vi "pci-6713-6025E-6733(set all analog).vi"(4 "6221 Control":dbl[](array[numeric])=[6.5, 7.0], 5 "Change 6221?":bool, 6 "6733 Control":sgl[](array[numeric])=[8.0, 3.0, 4.0, 0.0, 0.0, 6.46, 6.98, 0.0] format="%.3f", 7 "Change 6733":bool, 8 "6713 Control":sgl[](array[numeric])=[4.6, 0.5, 0.035, 7.35, 10.0, 4.0, 4.0, 2.703] format="%.3f", 9 "Change 6713?":bool=TRUE) -> (0 "Voltage limit (+-10V)":string[](array[string])=["OK ", "OK ", "OK ", "OK ", "OK ", "OK ", "OK ", "OK "], 1 "6733 Status":string="PCI-6733 OK", 2 "Voltage limit (+-10V)":string[](array[string])=["OK ", "OK ", "OK ", "OK ", "OK ", "OK ", "OK ", "OK "], 3 "6713 Status":string="PCI-6713 OK")   [LabVIEW 2013]
uses:
  AO Update Channel (scaled value).vi
  Instance           4 43Saved   pci-6713-6025E-6733(set all analog) .vi
  Instance           5 43Saved   pci-6713-6025E-6733(set all analog) .vi
  <vilib>/DAQmx/write.llb/DAQmx Write (Analog DBL 1Chan 1Samp).vi
panel:
  in  "Case Constant\n(See Context Help) 4":bool
  in  "Case Constant\n(See Context Help) 3":bool
  in  "Case Constant\n(See Context Help) 2":bool
  in  "Change 6025?":bool
  in  "Case Constant\n(See Context Help)":bool
  out "6733 Status 2":string="PCI-6733 OK"
  in  "6733 Control 2":sgl[](array[numeric])=[8.0, 3.0, 4.0, 0.0, 0.0, 6.46, 6.98, 0.0] format="%.3f"
  out "Voltage limit (+-10V) 2":string[](array[string])=["OK ", "OK ", "OK ", "OK ", "OK ", "OK ", "OK ", "OK "]
  out "Array 3":sgl[](array[numeric])=[8.0, 3.0, 4.0, 0.0, 0.0, 6.46, 6.98, 0.0]
  out "error out":errorcluster
  in  "Change 87Sr 6733":bool
  in  "87Sr 6733 Control":sgl[](array[numeric])=[8.0, 3.0, 4.0, 0.0, 0.0, 6.46, 6.98, 0.0] format="%.3f"
  out "87Sr Voltage limit (+-10V)":string[](array[string])=["OK ", "OK ", "OK ", "OK ", "OK ", "OK ", "OK ", "OK "]
  out "Array 2":sgl[](array[numeric])=[8.0, 3.0, 4.0, 0.0, 0.0, 6.46, 6.98, 0.0]
  out "Array":sgl[](array[numeric])=[8.0, 3.0, 4.0, 0.0, 0.0, 6.46, 6.98, 0.0]
  out "Voltage Limit (":string[](array[string])=["OK ", "OK "]
  in  "6025 Control":sgl[](array[numeric])=[-0.15, 0.1] format="%.3f"
  out "6025 Status":string="PCI-6025E OK"
  # "0..satabs offset for imaging"
  # "1... MOT power"
  # "2....MOT Jump Power"
  # "3....GENERAL PARAMETER: PAS AOM"
  # "4... GenPAram: offset lock"
  # "5....Vset for Lambda (0 to 10V)(pos for FET lock)"
  # "The DC supply\nvoltage for the\nZOS was 14.1 V"
  # "6....satabs offset for MOT"
  # "7.... satabs offset for cooling"
  # "0.....422 image AOM"
  # "PCI-6025E is NOT functional for Neutral Atoms.\nIt has been disabled in the block diagram, so\nchanging any of these values will not affect \nanything."
  # "1.....openr"
  # "Right now, put in units of \nvolts.  Freq to voltage \nconversion later."
  # "0.....100MHz Red MOT AOM (ZOS100) MHZ"
  # "1..... Power Control on  Red MOT AOM 5V full"
  # "dimage1 6.46V = 51.81MHz"
  # "dmot 6.980V = 35.50MHz"
  # "0.. Image AOM VCO (5V=41.5)"
  # "0..MOT AOM VCO (5V=41.5)"
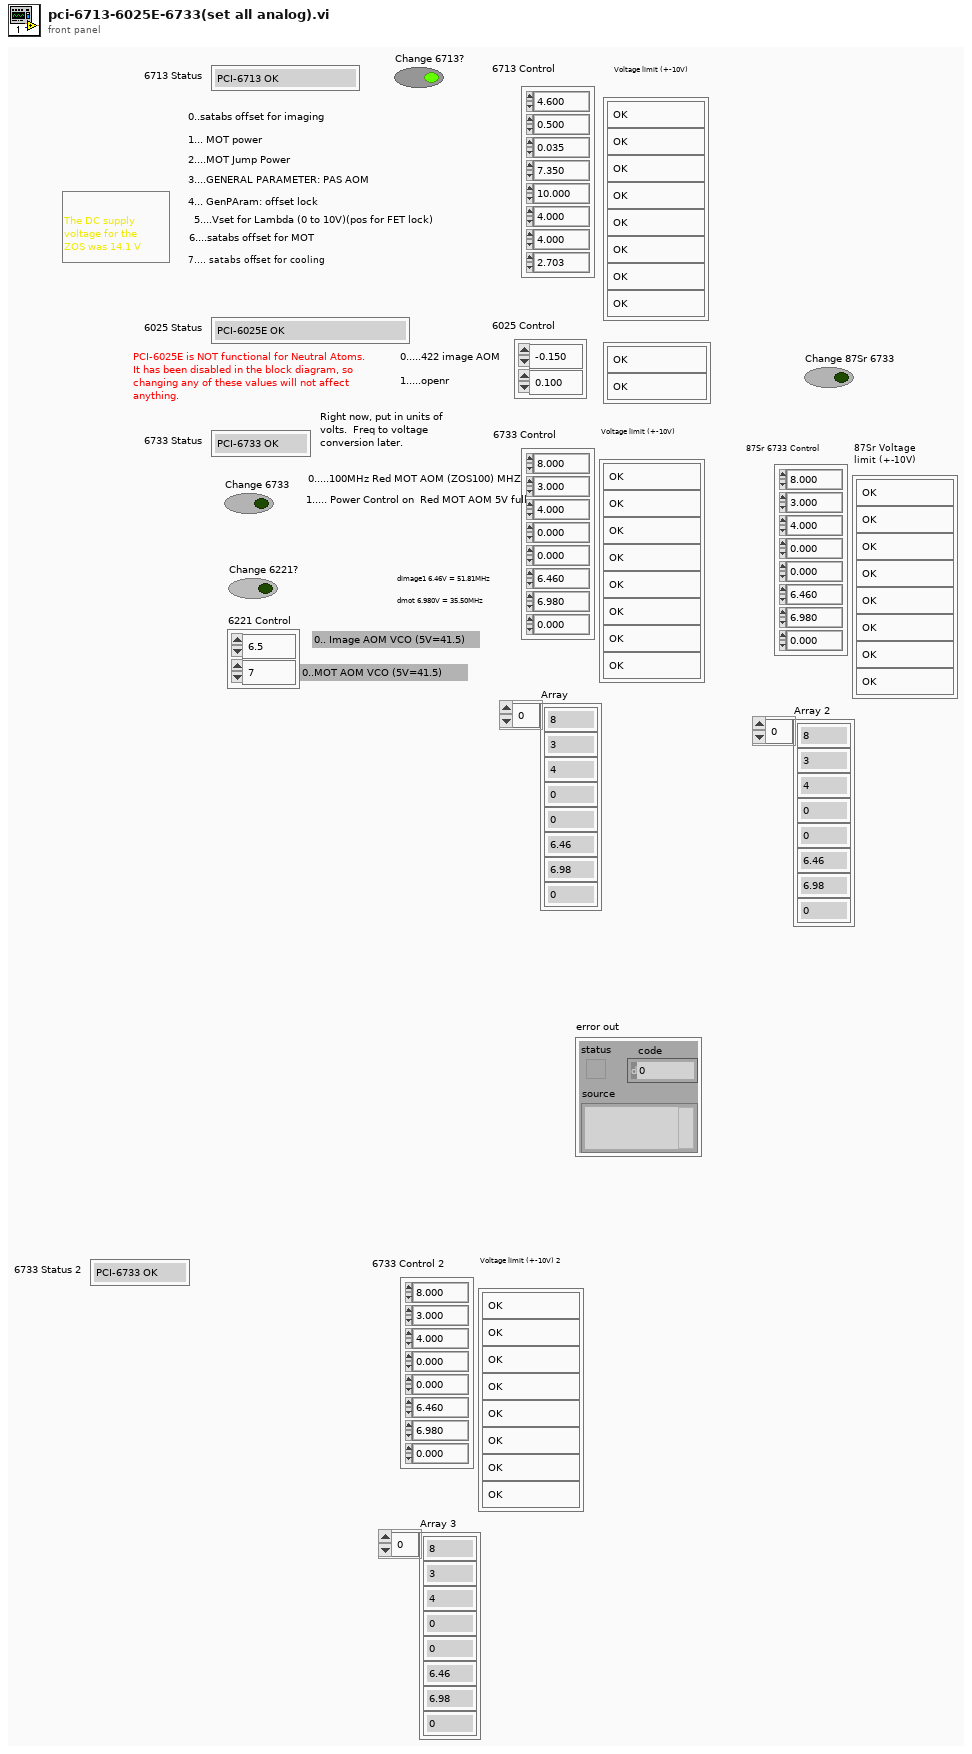
[diagram p1: front panel]
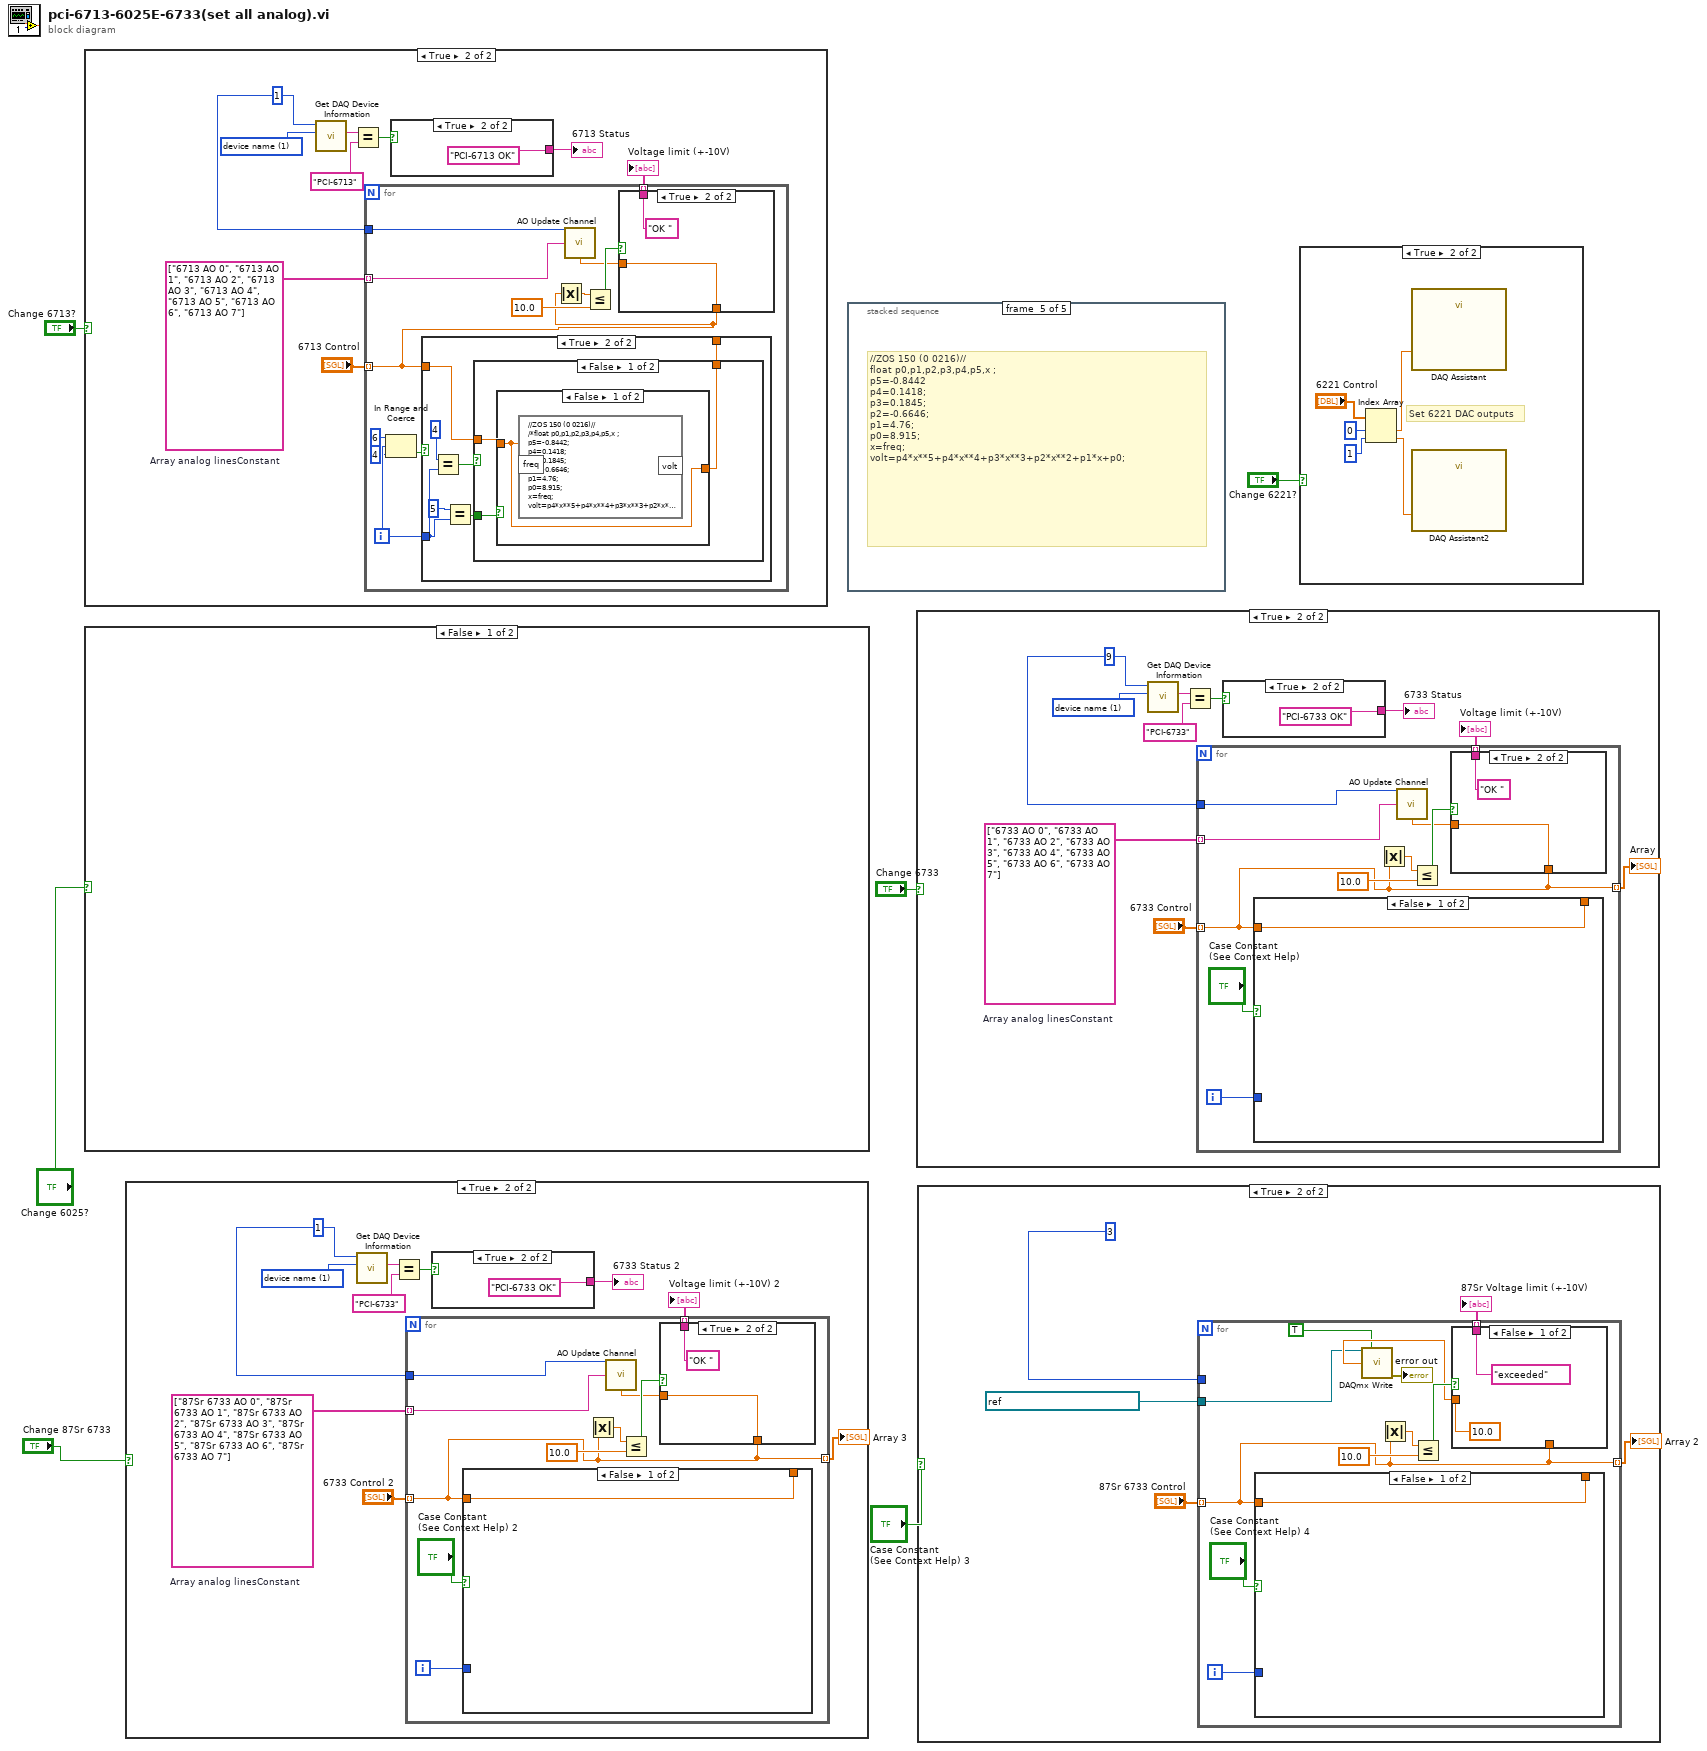
[diagram p0: block diagram]
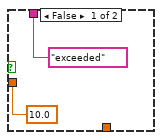
[diagram p3: hidden frame]
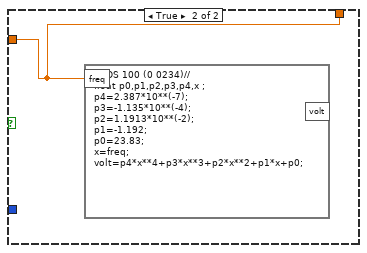
[diagram p4: hidden frame]
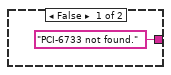
[diagram p5: hidden frame]
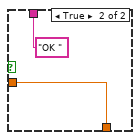
[diagram p7: hidden frame]
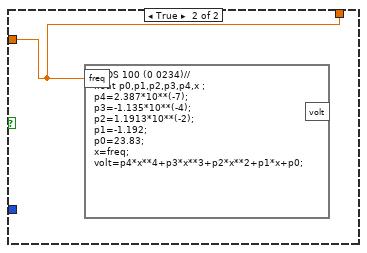
[diagram p8: hidden frame]
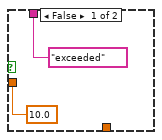
[diagram p11: hidden frame]
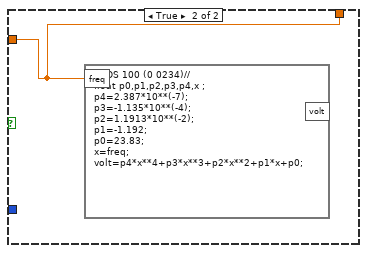
[diagram p12: hidden frame]
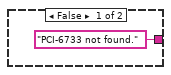
[diagram p13: hidden frame]
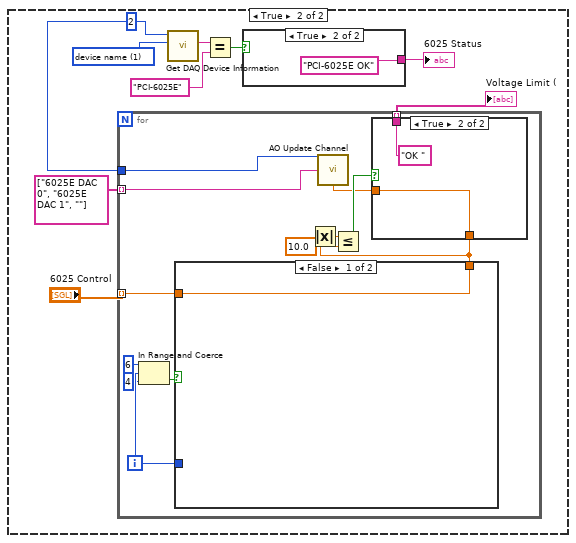
[diagram p14: hidden frame]
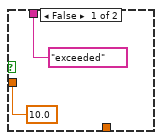
[diagram p15: hidden frame]
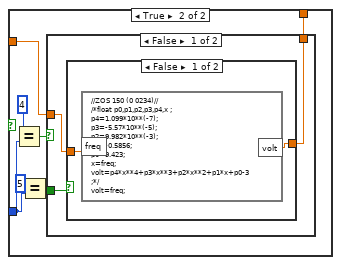
[diagram p16: hidden frame]
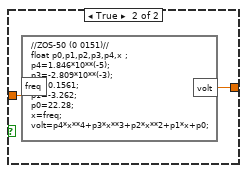
[diagram p17: hidden frame]
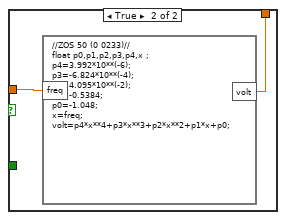
[diagram p18: hidden frame]
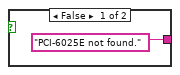
[diagram p19: hidden frame]
diagram:
  n1 = case shown="True" "Change 6713?" {
    frame False {
    }
    frame True {
      w7 = tag[] ["6713 AO 0", "6713 AO 1", "6713 AO 2", "6713 AO 3", "6713 AO 4", "6713 AO 5", "6713 AO 6", "6713 AO 7"]  # Array analog linesConstant
      w15 = u32 1 items=["NI-DAQ version", "device name", "base address", "data transfer mode for analog input", "data transfer mode for analog output group 1", "data transfer mode for analog output group 2", "data transfer mode for GPCTR 0", "data transfer mode for GPCTR 1", "data transfer mode for digital I/O group 1", "data transfer mode for digital I/O group 2", "device type code", "DMA A level", "DMA B level", "DMA C level", "interrupt A level", "interrupt B level", "reserved", "lpt device mode", "DAQCard-700 counter 1 source", "interrupt generation mode", "device state during suspend mode", "computer name", "serial number", "counter type"] ("information type")
      w10 = u32 1 ("task ID or device")
      n2 = call "Get DAQ Device Information.vi"("information type"=w15, "task ID or device"=w10) -> ("information string"=w14:string)  [unwired: 7 in, 2 out]
      n3 = Equal?(x=w14, y="PCI-6713") -> (x = y?=w12:bool)
      n4 = for {
        tunnel: w10 -> [w27]
        tunnel: "6713 Control" -> [w16] mode=indexing
        tunnel: w7 -> [w26] mode=indexing
        tunnel: [w17] -> w8 mode=indexing
        i -> [w25]
        n5 = In Range and Coerce(upper limit=6, x=w25, lower limit=4) -> (In Range?=w22:bool)  [unwired: 1 out]
        n6 = case shown="True" w22 {
          tunnel: w16 -> [w32 w34]
          tunnel: [w32 w33] -> _
          tunnel: w25 -> [_ w37]
          frame False {
          }
          frame True {
            n7 = Equal?(x=4, y=w37) -> (x = y?=w38:bool)
            n8 = Equal?(x=5, y=w37) -> (x = y?=w35:bool)
            n9 = case shown="False" w38 {
              tunnel: w35 -> [w42 _]
              tunnel: w34 -> [w41 w46]
              tunnel: [w40 w46] -> w33
              frame False {
                n10 = case shown="False" w42 {
                  tunnel: w41 -> [w43 w45]
                  tunnel: [w43 w44] -> w40
                  frame False {
                    n11 = formula code="//ZOS 150 (0 0216)//\n/*float p0,p1,p2,p3,p4,p5,x ;\np5=-0.8442;\np4=0.1418;\np3=0.1845;\np2=-0.6646;\np1=4.76;\np0=8.915;\nx=freq;\nvolt=p4*x**5+p4*x**4+p3*x**3+p2*x**2+p1*x+p0;\n*/\nvolt=freq;"("freq"=w43) -> ()  [unwired: 1 out]
                  }
                  frame True {
                    n12 = formula code="//ZOS 100 (0 0214)//\nfloat p0,p1,p2,p3,p4,x ;\np4=6.457*10**(-7);\np3=-2.117*10**(-4);\np2=2.473*10**(-2);\np1=-0.9844;\np0=11.55;\nx=freq;\nvolt=p4*x**4+p3*x**3+p2*x**2+p1*x+p0;"("freq"=w45) -> ("volt"=w44:dbl)
                  }
                }
              }
              frame True {
                n13 = formula code="//ZOS 150 (0 0234)//\nfloat p0,p1,p2,p3,p4,x ;\np4=1.099*10**(-7);\np3=-5.57*10**(-5);\np2=9.982*10**(-3);\np1=-0.5866;\np0=9.423;\nx=freq;\nvolt=p4*x**4+p3*x**3+p2*x**2+p1*x+p0;"("freq"=w46) -> ()  [unwired: 1 out]
              }
            }
          }
        }
        n14 = Absolute Value(x=w16) -> (abs(x)=w21:sgl)
        n15 = Less Or Equal?(x=w21, y=10.0) -> (x <= y?=w19:bool)
        n16 = case shown="True" w19 {
          tunnel: w16 -> [_ w31]
          tunnel: [10.0 w31] -> w18
          tunnel: ["exceeded" ("String") "OK " ("String")] -> w17
          frame False {
          }
          frame True {
          }
        }
        n17 = call-poly "AO Update Channel.vi"("value"=w18, "channel (0)"=w26, "device"=w27) -> ()
      }
      "Voltage limit (+-10V)" <- w8
      n18 = case shown="True" w12 {
        tunnel: ["PCI-6713 not found." "PCI-6713 OK"] -> w11
        frame False {
        }
        frame True {
        }
      }
      "6713 Status" <- w11
    }
  }
  n19 = case shown="False" "Change 6025?" {
    frame False {
    }
    frame True {
      w57 = u32 1 items=["NI-DAQ version", "device name", "base address", "data transfer mode for analog input", "data transfer mode for analog output group 1", "data transfer mode for analog output group 2", "data transfer mode for GPCTR 0", "data transfer mode for GPCTR 1", "data transfer mode for digital I/O group 1", "data transfer mode for digital I/O group 2", "device type code", "DMA A level", "DMA B level", "DMA C level", "interrupt A level", "interrupt B level", "reserved", "lpt device mode", "DAQCard-700 counter 1 source", "interrupt generation mode", "device state during suspend mode", "computer name", "serial number", "counter type"] ("information type")
      w52 = u32 2 ("task ID or device")
      n20 = for {
        tunnel: w52 -> [w70]
        tunnel: "6025 Control" -> [w64] mode=indexing
        tunnel: tag[] ["6025E DAC 0", "6025E DAC 1", ""] ("Array analog linesConstant") -> [w69] mode=indexing
        tunnel: [w58] -> w50 mode=indexing
        i -> [w68]
        n21 = In Range and Coerce(upper limit=6, x=w68, lower limit=4) -> (In Range?=w65:bool)  [unwired: 1 out]
        n22 = case shown="False" w65 {
          tunnel: w64 -> [w75 w77]
          tunnel: [w75 w76] -> w63
          tunnel: w68 -> [_ w80]
          frame False {
          }
          frame True {
            n23 = Equal?(x=4, y=w80) -> (x = y?=w81:bool)
            n24 = Equal?(x=5, y=w80) -> (x = y?=w78:bool)
            n25 = case shown="False" w81 {
              tunnel: w78 -> [w85 _]
              tunnel: w77 -> [w84 w91]
              tunnel: [w83 w90] -> w76
              frame False {
                n26 = case shown="False" w85 {
                  tunnel: w84 -> [w87 w89]
                  tunnel: [w86 w88] -> w83
                  frame False {
                    n27 = formula code="//ZOS 150 (0 0234)//\n/*float p0,p1,p2,p3,p4,x ;\np4=1.099*10**(-7);\np3=-5.57*10**(-5);\np2=9.982*10**(-3);\np1=-0.5856;\np0=9.423;\nx=freq;\nvolt=p4*x**4+p3*x**3+p2*x**2+p1*x+p0-3\n;*/\nvolt=freq;"("freq"=w87) -> ("volt"=w86:dbl)
                  }
                  frame True {
                    n28 = formula code="//ZOS-50 (0 0151)//\nfloat p0,p1,p2,p3,p4,x ;\np4=1.846*10**(-5);\np3=-2.809*10**(-3);\np2=0.1561;\np1=-3.262;\np0=22.28;\nx=freq;\nvolt=p4*x**4+p3*x**3+p2*x**2+p1*x+p0;"("freq"=w89) -> ("volt"=w88:dbl)
                  }
                }
              }
              frame True {
                n29 = formula code="//ZOS 50 (0 0233)//\nfloat p0,p1,p2,p3,p4,x ;\np4=3.992*10**(-6);\np3=-6.824*10**(-4);\np2=4.095*10**(-2);\np1=-0.5384;\np0=-1.048;\nx=freq;\nvolt=p4*x**4+p3*x**3+p2*x**2+p1*x+p0;"("freq"=w91) -> ("volt"=w90:dbl)
              }
            }
          }
        }
        n30 = Absolute Value(x=w63) -> (abs(x)=w62:dbl)
        n31 = Less Or Equal?(x=w62, y=10.0) -> (x <= y?=w60:bool)
        n32 = case shown="True" w60 {
          tunnel: w63 -> [_ w74]
          tunnel: [10.0 w74] -> w59
          tunnel: ["exceeded" ("String") "OK " ("String")] -> w58
          frame False {
          }
          frame True {
          }
        }
        n33 = call-poly "AO Update Channel.vi"("value"=w59, "channel (0)"=w69, "device"=w70) -> ()
      }
      "Voltage Limit (" <- w50
      n34 = call "Get DAQ Device Information.vi"("information type"=w57, "task ID or device"=w52) -> ("information string"=w56:string)  [unwired: 7 in, 2 out]
      n35 = Equal?(x=w56, y="PCI-6025E") -> (x = y?=w54:bool)
      n36 = case shown="True" w54 {
        tunnel: ["PCI-6025E not found." "PCI-6025E OK"] -> w53
        frame False {
        }
        frame True {
        }
      }
      "6025 Status" <- w53
    }
  }
  n37 = case shown="True" "Change 87Sr 6733" {
    frame False {
    }
    frame True {
      w95 = tag[] ["87Sr 6733 AO 0", "87Sr 6733 AO 1", "87Sr 6733 AO 2", "87Sr 6733 AO 3", "87Sr 6733 AO 4", "87Sr 6733 AO 5", "87Sr 6733 AO 6", "87Sr 6733 AO 7"]  # Array analog linesConstant
      w103 = u32 1 items=["NI-DAQ version", "device name", "base address", "data transfer mode for analog input", "data transfer mode for analog output group 1", "data transfer mode for analog output group 2", "data transfer mode for GPCTR 0", "data transfer mode for GPCTR 1", "data transfer mode for digital I/O group 1", "data transfer mode for digital I/O group 2", "device type code", "DMA A level", "DMA B level", "DMA C level", "interrupt A level", "interrupt B level", "reserved", "lpt device mode", "DAQCard-700 counter 1 source", "interrupt generation mode", "device state during suspend mode", "computer name", "serial number", "counter type"] ("information type")
      w98 = u32 1 ("task ID or device")
      n38 = call "Get DAQ Device Information.vi"("information type"=w103, "task ID or device"=w98) -> ("information string"=w102:string)  [unwired: 7 in, 2 out]
      n39 = Equal?(x=w102, y="PCI-6733") -> (x = y?=w100:bool)
      n40 = for {
        tunnel: w98 -> [w113]
        tunnel: "6733 Control 2" -> [w104] mode=indexing
        tunnel: w95 -> [w112] mode=indexing
        tunnel: [w107] -> w96 mode=indexing
        tunnel: [w104] -> w94 mode=indexing
        i -> [w106]
        n41 = case shown="False" "Case Constant\n(See Context Help) 2" {
          tunnel: w104 -> [w118 w119]
          tunnel: [w118 w119] -> _
          tunnel: w106 -> [_ _]
          frame False {
          }
          frame True {
            n42 = formula code="//ZOS 100 (0 0234)//\nfloat p0,p1,p2,p3,p4,x ;\np4=2.387*10**(-7);\np3=-1.135*10**(-4);\np2=1.1913*10**(-2);\np1=-1.192;\np0=23.83;\nx=freq;\nvolt=p4*x**4+p3*x**3+p2*x**2+p1*x+p0;"("freq"=w119) -> ()  [unwired: 1 out]
          }
        }
        n43 = Absolute Value(x=w104) -> (abs(x)=w111:sgl)
        n44 = Less Or Equal?(x=w111, y=10.0) -> (x <= y?=w109:bool)
        n45 = case shown="True" w109 {
          tunnel: w104 -> [_ w117]
          tunnel: [10.0 w117] -> w108
          tunnel: ["exceeded" ("String") "OK " ("String")] -> w107
          frame False {
          }
          frame True {
          }
        }
        n46 = call-poly "AO Update Channel.vi"("value"=w108, "channel (0)"=w112, "device"=w113) -> ()
      }
      "Voltage limit (+-10V) 2" <- w96
      "Array 3" <- w94
      n47 = case shown="True" w100 {
        tunnel: ["PCI-6733 not found." "PCI-6733 OK"] -> w99
        frame False {
        }
        frame True {
        }
      }
      "6733 Status 2" <- w99
    }
  }
  n48 = stacked-sequence {
    frame #0 {
      # "//ZOS-50 (0 0151)//\nfloat p0,p1,p2,p3,p4,x ;\np4=1.846*10**(-5);\np3=-2.809*10**(-3);\np2=0.1561;\np1=-3.262;\np0=22.28;\nx=freq;\nvolt=p4*x**4+p3*x**3+p2*x**2+p1*x+p0;"
    }
    frame #1 {
      # "//ZOS 100 (0 0214)//\nfloat p0,p1,p2,p3,p4,x ;\np4=6.457*10**(-7);\np3=-2.117*10**(-4);\np2=2.473*10**(-2);\np1=-0.9844;\np0=11.55;\nx=freq;\nvolt=p4*x**4+p3*x**3+p2*x**2+p1*x+p0;"
    }
    frame #2 {
      # "//ZOS 150 (0 0234)//\nfloat p0,p1,p2,p3,p4,x ;\np4=1.099*10**(-7);\np3=-5.57*10**(-5);\np2=9.982*10**(-3);\np1=-0.5866;\np0=9.423;\nx=freq;\nvolt=p4*x**4+p3*x**3+p2*x**2+p1*x+p0;"
    }
    frame #3 {
      # "//ZOS 50 (0 0233)//\nfloat p0,p1,p2,p3,p4,x ;\np4=3.992*10**(-6);\np3=-6.824*10**(-4);\np2=4.095*10**(-2);\np1=-0.5384;\np0=-1.048;\nx=freq;\nvolt=p4*x**4+p3*x**3+p2*x**2+p1*x+p0;"
    }
    frame #4 {
      # "//ZOS 150 (0 0216)//\nfloat p0,p1,p2,p3,p4,p5,x ;\np5=-0.8442\np4=0.1418;\np3=0.1845;\np2=-0.6646;\np1=4.76;\np0=8.915;\nx=freq;\nvolt=p4*x**5+p4*x**4+p3*x**3+p2*x**2+p1*x+p0;"
    }
  }
  n49 = case shown="True" "Change 6733" {
    frame False {
    }
    frame True {
      w123 = tag[] ["6733 AO 0", "6733 AO 1", "6733 AO 2", "6733 AO 3", "6733 AO 4", "6733 AO 5", "6733 AO 6", "6733 AO 7"]  # Array analog linesConstant
      w131 = u32 1 items=["NI-DAQ version", "device name", "base address", "data transfer mode for analog input", "data transfer mode for analog output group 1", "data transfer mode for analog output group 2", "data transfer mode for GPCTR 0", "data transfer mode for GPCTR 1", "data transfer mode for digital I/O group 1", "data transfer mode for digital I/O group 2", "device type code", "DMA A level", "DMA B level", "DMA C level", "interrupt A level", "interrupt B level", "reserved", "lpt device mode", "DAQCard-700 counter 1 source", "interrupt generation mode", "device state during suspend mode", "computer name", "serial number", "counter type"] ("information type")
      w126 = u32 9 ("task ID or device")
      n50 = call "Get DAQ Device Information.vi"("information type"=w131, "task ID or device"=w126) -> ("information string"=w130:string)  [unwired: 7 in, 2 out]
      n51 = Equal?(x=w130, y="PCI-6733") -> (x = y?=w128:bool)
      n52 = for {
        tunnel: w126 -> [w141]
        tunnel: "6733 Control" -> [w132] mode=indexing
        tunnel: w123 -> [w140] mode=indexing
        tunnel: [w135] -> w124 mode=indexing
        tunnel: [w132] -> w122 mode=indexing
        i -> [w134]
        n53 = case shown="False" "Case Constant\n(See Context Help)" {
          tunnel: w132 -> [w146 w147]
          tunnel: [w146 w147] -> _
          tunnel: w134 -> [_ _]
          frame False {
          }
          frame True {
            n54 = formula code="//ZOS 100 (0 0234)//\nfloat p0,p1,p2,p3,p4,x ;\np4=2.387*10**(-7);\np3=-1.135*10**(-4);\np2=1.1913*10**(-2);\np1=-1.192;\np0=23.83;\nx=freq;\nvolt=p4*x**4+p3*x**3+p2*x**2+p1*x+p0;"("freq"=w147) -> ()  [unwired: 1 out]
          }
        }
        n55 = Absolute Value(x=w132) -> (abs(x)=w139:sgl)
        n56 = Less Or Equal?(x=w139, y=10.0) -> (x <= y?=w137:bool)
        n57 = case shown="True" w137 {
          tunnel: w132 -> [_ w145]
          tunnel: [10.0 w145] -> w136
          tunnel: ["exceeded" ("String") "OK " ("String")] -> w135
          frame False {
          }
          frame True {
          }
        }
        n58 = call-poly "AO Update Channel.vi"("value"=w136, "channel (0)"=w140, "device"=w141) -> ()
      }
      "Voltage limit (+-10V)" <- w124
      "Array" <- w122
      n59 = case shown="True" w128 {
        tunnel: ["PCI-6733 not found." "PCI-6733 OK"] -> w127
        frame False {
        }
        frame True {
        }
      }
      "6733 Status" <- w127
    }
  }
  n60 = case shown="True" "Case Constant\n(See Context Help) 3" {
    frame False {
    }
    frame True {
      n61 = for {
        tunnel: u32 3 ("task ID or device") -> [_]
        tunnel: "87Sr 6733 Control" -> [w159] mode=indexing
        tunnel: [w162] -> w152 mode=indexing
        tunnel: [w159] -> w151 mode=indexing
        tunnel: refnum<k21> "Red MOT Arbitrary Waveform Sr87" ("task/channels in") -> [w157]
        i -> [w161]
        n62 = case shown="False" "Case Constant\n(See Context Help) 4" {
          tunnel: w159 -> [w170 w171]
          tunnel: [w170 w171] -> _
          tunnel: w161 -> [_ _]
          frame False {
          }
          frame True {
            n63 = formula code="//ZOS 100 (0 0234)//\nfloat p0,p1,p2,p3,p4,x ;\np4=2.387*10**(-7);\np3=-1.135*10**(-4);\np2=1.1913*10**(-2);\np1=-1.192;\np0=23.83;\nx=freq;\nvolt=p4*x**4+p3*x**3+p2*x**2+p1*x+p0;"("freq"=w171) -> ()  [unwired: 1 out]
          }
        }
        n64 = Absolute Value(x=w159) -> (abs(x)=w165:sgl)
        n65 = Less Or Equal?(x=w165, y=10.0) -> (x <= y?=w163:bool)
        n66 = case shown="False" w163 {
          tunnel: w159 -> [_ w169]
          tunnel: [10.0 w169] -> w158
          tunnel: ["exceeded" ("String") "OK " ("String")] -> w162
          frame False {
          }
          frame True {
          }
        }
        n67 = call-poly <vilib>:"DAQmx Write.vi"("task/channels in"=w157, "auto start"=TRUE, "data"=w158) -> ("error out"=→"error out":errorcluster)  [unwired: 10 in, 2 out]
      }
      "87Sr Voltage limit (+-10V)" <- w152
      "Array 2" <- w151
    }
  }
  n68 = case shown="True" "Change 6221?" {
    frame False {
    }
    frame True {
      # "Set 6221 DAC outputs"
      n69 = Index Array(array="6221 Control", index #1=0 ("index"), index #2=1 ("index")) -> (element #1=w173:dbl, element #2=w172:dbl)
      n70 = call "DAQ Assistant"("data"=w173) -> ()  [unwired: 9 in, 2 out]
      n71 = call "DAQ Assistant2"("data"=w172) -> ()  [unwired: 9 in, 2 out]
    }
  }
